vi "STOP_GLOBAL.vi"() -> ()   [LabVIEW 2022 SP3]
panel:
  in  "ALL STOP":bool
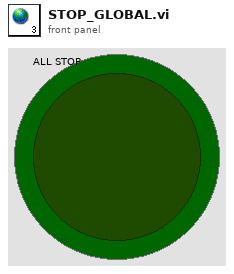
[diagram p1: front panel]
diagram:
